vi "Configure Setpoint.vi"(8 "error in (no error)":errorcluster, 9 "Setpoint (0.00000E+0)":dbl min=0.0 max=100000000.0 step=1e-06 format="%^.5e", 10 "Output (0: Sample Heater)":u16(ring) items=["Sample Heater", "Warm-up Heater (output 1)"], 11 "VISA resource name":refnum<visa-resource-name>) -> (0 "error out":errorcluster, 3 "VISA resource name out":refnum<visa-resource-name>)   [LabVIEW 2018, in "Lake Shore 372.lvlib"]
doc: "Configures the temperature control setpoint in preferred units. \nSee Model 372 manual for further explanation."
uses:
  Lake Shore 372.lvlib
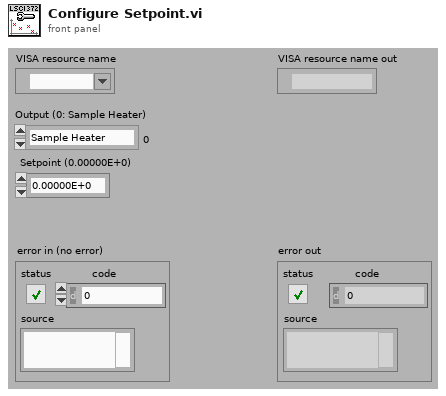
[diagram p1: front panel]
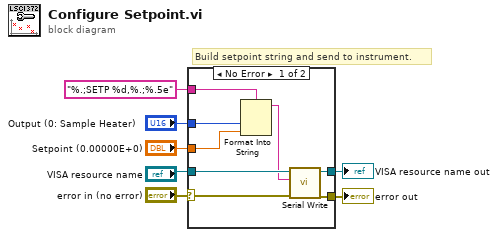
[diagram p0: block diagram]
diagram:
  # "Build setpoint string and send to instrument."
  n1 = case shown="No Error" "error in (no error)" {
    selector: "error in (no error)" -> [w8 w16]
    tunnel: "%.;SETP %d,%.;%.5e" -> [w15 _]
    tunnel: [w14 w17] -> w6
    tunnel: [w13 w16] -> w5
    tunnel: "VISA resource name" -> [w12 w17]
    tunnel: "Setpoint (0.00000E+0)" -> [w11 _]
    tunnel: "Output (0: Sample Heater)" -> [w9 _]
    frame No Error {
      n2 = Format Into String(format string=w15, w9, w11) -> (resulting string=w10:string)  [unwired: 2 in, 1 out]
      n3 = call "Serial Write.vi"("error in (no error)"=w8, "Write Buffer (\"\")"=w10, "VISA resource name"=w12) -> ("error out"=w13:errorcluster, "VISA resource name out"=w14:refnum<visa-resource-name>)  [unwired: 6 in, 1 out]
    }
    frame Error {
    }
  }
  "error out" <- w5
  "VISA resource name out" <- w6
